vi "Endurance Reset Operation.vi"(8 "error in (no error)":errorcluster, 9 "SLV":dbl=2.8 format="%#_13g", 10 "WLV":dbl=4.0 format="%#_13g", 11 "instrument handle":refnum<k15>="PXI1Slot2 (123)") -> (0 "error out":errorcluster, 3 "instrument handle out":refnum<k15>="PXI1Slot2 (123)")   [LabVIEW 2018]
uses:
  <instrlib>/niDigital/niDigital.llb/niDigital Burst Pattern (Burst Only).vi
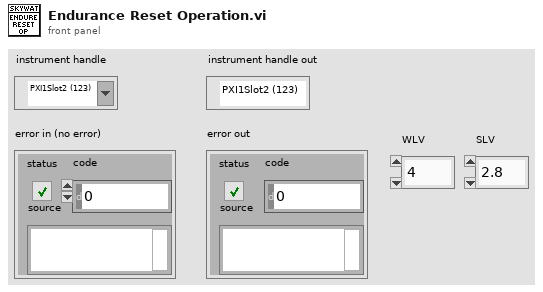
[diagram p1: front panel]
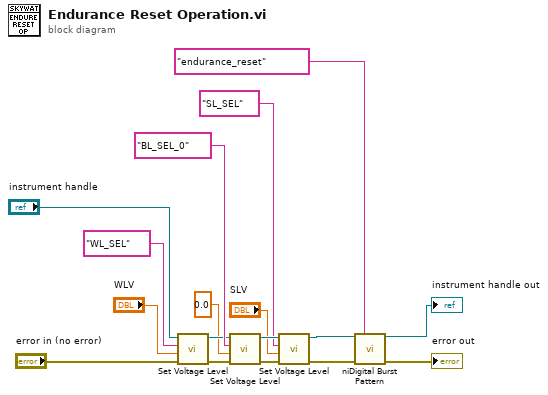
[diagram p0: block diagram]
diagram:
  n1 = call "Set Voltage Level.vi"("error in (no error)"="error in (no error)", "level (V)"="WLV", "channel list"="WL_SEL", "instrument handle"="instrument handle") -> ("error out"=w11:errorcluster, "instrument handle out"=w12:refnum<k15>)  [unwired: 6 in]
  n2 = call "Set Voltage Level.vi"("error in (no error)"=w11, "level (V)"=0.0, "channel list"="BL_SEL_0", "instrument handle"=w12) -> ("error out"=w10:errorcluster, "instrument handle out"=w13:refnum<k15>)  [unwired: 6 in]
  n3 = call "Set Voltage Level.vi"("error in (no error)"=w10, "level (V)"="SLV", "channel list"="SL_SEL", "instrument handle"=w13) -> ("error out"=w3:errorcluster, "instrument handle out"=w5:refnum<k15>)  [unwired: 6 in]
  n4 = call-poly <instrlib>:"niDigital Burst Pattern.vi"("instrument handle"=w5, "start label"="endurance_reset", "error in"=w3) -> ("instrument handle out"=→"instrument handle out":refnum<k15>, "error out"=→"error out":errorcluster)  [unwired: 11 in]
